vi "Manual VIP Prebuild.vi"() -> ()   [LabVIEW 2020]
uses:
  dev/Tags.ctl
panel:
  out "Next Version":string
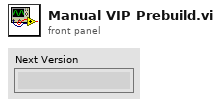
[diagram p1: front panel]
types:
  T1 = typedef "Tags.ctl" = enum16{"sol.squarebattle.version"}
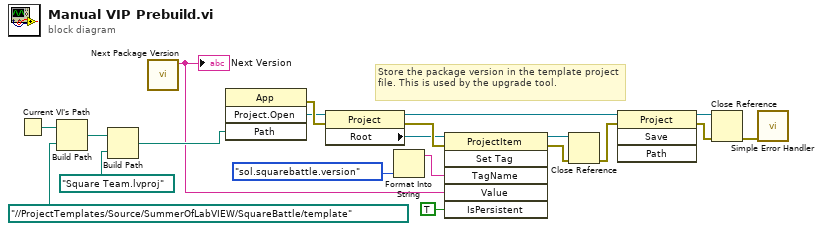
[diagram p0: block diagram]
diagram:
  # "Store the package version in the template project file. This is used by the upgrade tool."
  n1 = Current VI's Path() -> (path=w20:path)
  n2 = Build Path(base path=w20, name or relative path=path "../../ProjectTemplates/Source/SummerOfLabVIEW/SquareBattle/template") -> (appended path=w3:path)
  n3 = Build Path(base path=w3, name or relative path=path "Square Team.lvproj") -> (appended path=w6:path)
  n4 = call "Next Package Version.vi"() -> ("Next Version"=w1:string)  [unwired: 10 in, 1 out]
  "Next Version" <- w1
  n5 = invoke class="App" method="Project.Open"("Path"=w6) -> (error out=w18:errorcluster, "Project:Open"=w15:refnum<vi>)  [unwired: 3 in, 2 out]
  n6 = property class="Project"(reference=w15, error in=w18) -> (reference out=w16:refnum<vi>, error out=w17:errorcluster, "Root"=w14:refnum<vi>)
  n7 = Format Into String(Tags."sol.squarebattle.version" ("Tags")) -> (resulting string=w4:string)  [unwired: 3 in, 1 out]
  n8 = invoke class="ProjectItem" method="Set Tag"(reference=w14, error in=w17, "TagName"=w4, "Value"=w1, "IsPersistent"=TRUE ("Is Persistent (T)")) -> (reference out=w12:refnum<vi>, error out=w11:errorcluster)  [unwired: 1 in, 4 out]
  n9 = Close Reference(reference=w12, error in (no error)=w11) -> (error out=w10:errorcluster)
  n10 = invoke class="Project" method="Save"(reference=w16, error in=w10) -> (reference out=w9:refnum<vi>, error out=w8:errorcluster)  [unwired: 2 in, 2 out]
  n11 = Close Reference(reference=w9, error in (no error)=w8) -> (error out=w7:errorcluster)
  n12 = call <vilib>:"Simple Error Handler.vi"("error in (no error)"=w7) -> ()  [unwired: 4 in, 5 out]
